vi "DHE_GetAppendID.vi"() -> (7 "DHE_asyncexp":bool)   [LabVIEW 2016]
uses:
  private/vis/DHE_VarAction.ctl
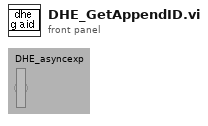
[diagram p1: front panel]
types:
  T1 = typedef "DHE_VarAction.ctl" = enum16{"read", "write"}
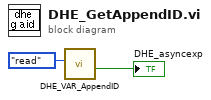
[diagram p0: block diagram]
diagram:
  n1 = call "DHE_VAR_AppendID.vi"("action"=DHE_VarAction."read") -> ("appendobsid"=→"DHE_asyncexp":bool)  [unwired: 1 in, 9 out]
